vi "Read Pixels and Copy to Display Image New.vi"(0 "fpga interface in":refnum<k20>, 5 "display channel number":i32, 7 "serial channel display parameters":T6[](array[typedef]) {"RAW parameters"."bayer parameters"."blue gain" format="%_4g"; "RAW parameters"."bayer parameters"."green gain" format="%_4g"; "RAW parameters"."bayer parameters"."red gain" format="%_4g"; "RAW parameters"."bayer parameters"."algorithm" items=["Bilinear", "VNG"]; "RAW parameters"."bayer parameters"."pattern" items=["GB", "GR", "BG", "RG"]}, 9 "image metadata":T4, 11 "error in (no error)":errorcluster) -> (4 "fpga interface out":refnum<k20>, 6 "display image":T3, 8 "output cluster":T2, 15 "error out":errorcluster)   [LabVIEW 2026]
uses:
  Types/Serial Channel Display Parameters.ctl
  <vilib>/vision/Image Controls.llb/IMAQ Image.ctl
  Types/RAW Interpretation for Display.ctl
  FPGA/Common/Types/Image Metadata.ctl
  <instrlib>/FlexRIO/CSI-2/v2/Common/Types/LLP Data Type.ctl
  GettingStarted_Common_148X_Host.lvlib
  <instrlib>/FlexRIO/CSI-2/v2/Common/NI CSI-2 API Common v2.lvlib
  FPGA/Common/GettingStarted_Common_148X_FPGA.lvlib
panel:
  in  "Image Metadata and Data":T2 {"RAW parameters"."bayer parameters"."blue gain" format="%_4g"; "RAW parameters"."bayer parameters"."green gain" format="%_4g"; "RAW parameters"."bayer parameters"."red gain" format="%_4g"; "RAW parameters"."bayer parameters"."algorithm" items=["Bilinear", "VNG"]; "RAW parameters"."bayer parameters"."pattern" items=["GB", "GR", "BG", "RG"]}
  out "Array":u8[](array[numeric])
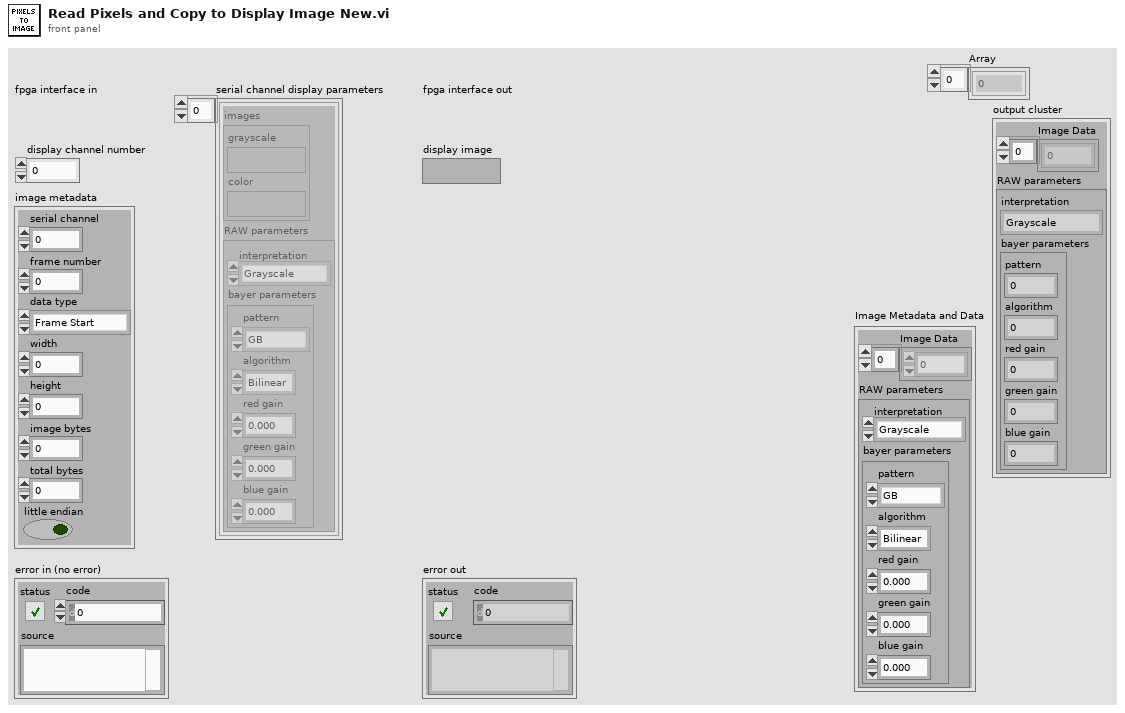
[diagram p1: front panel]
types:
  T1 = typedef "GettingStarted_Common_148X_Host.lvlib/RAW Interpretation for Display.ctl" = enum16{"Grayscale", "Bayer", "RGB", "YUV422", "YUV420", "Legacy YUV420"}
  T2 = cluster{"Image Data":u8[], "RAW parameters":cluster{"interpretation":T1, "bayer parameters":cluster{"pattern":i32, "algorithm":i32, "red gain":dbl, "green gain":dbl, "blue gain":dbl}}}
  T3 = typedef "IMAQ Image.ctl" = refnum<image>
  T4 = typedef "GettingStarted_Common_148X_FPGA.lvlib/Image Metadata.ctl" = cluster{"serial channel":fxp<+,3,3>, "frame number":u16, "data type":T5, "width":u16, "height":u16, "image bytes":u32, "total bytes":u32, "little endian":bool}
  T5 = typedef "NI CSI-2 API Common v2.lvlib/LLP Data Type.ctl" = enum8{"Frame Start", "Frame End", "Line Start", "Line End", "End of Transmission", "Reserved 0", "Reserved 1", "Reserved 2", "Generic Short Packet 1", "Generic Short Packet 2", "Generic Short Packet 3", "Generic Short Packet 4", "Generic Short Packet 5", "Generic Short Packet 6", "Generic Short Packet 7", "Generic Short Packet 8", "Null", "Blanking Data", "Embedded 8-bit non Image Data", "Generic Long Packet 1", "Generic Long Packet 2", "Generic Long Packet 3", "Generic Long Packet 4", "Reserved 3", "YUV420 8-bit", "YUV420 10-bit", "Legacy YUV420 8-bit", "Reserved 4", "YUV420 8-bit Chroma Shifted", "YUV420 10-bit Chroma Shifted", "YUV422 8-bit", "YUV422 10-bit", "RGB444", "RGB555", "RGB565", "RGB666", "RGB888", "Reserved 5", "Reserved 6", "RAW 24", "RAW 6", "RAW 7", "RAW 8", "RAW 10", "RAW 12", "RAW 14", "RAW 16", "RAW 20", "User Defined 8-bit Data 1", "User Defined 8-bit Data 2", "User Defined 8-bit Data 3", "User Defined 8-bit Data 4", "User Defined 8-bit Data 5", "User Defined 8-bit Data 6", "User Defined 8-bit Data 7", "User Defined 8-bit Data 8", "USL Command", "Reserved 7", "Reserved 8", "Reserved 9", "Reserved 10", "Reserved 11", "Reserved 12", "LRTE EPD Spacer"}
  T6 = typedef "GettingStarted_Common_148X_Host.lvlib/Serial Channel Display Parameters.ctl" = cluster{"images":cluster{"grayscale":T3, "color":T3}, "RAW parameters":cluster{"interpretation":T1, "bayer parameters":cluster{"pattern":i32, "algorithm":i32, "red gain":dbl, "green gain":dbl, "blue gain":dbl}}}
  T7 = cluster{"interpretation":T1, "bayer parameters":cluster{"pattern":i32, "algorithm":i32, "red gain":dbl, "green gain":dbl, "blue gain":dbl}}
  T8 = cluster{"pattern":i32, "algorithm":i32, "red gain":dbl, "green gain":dbl, "blue gain":dbl}
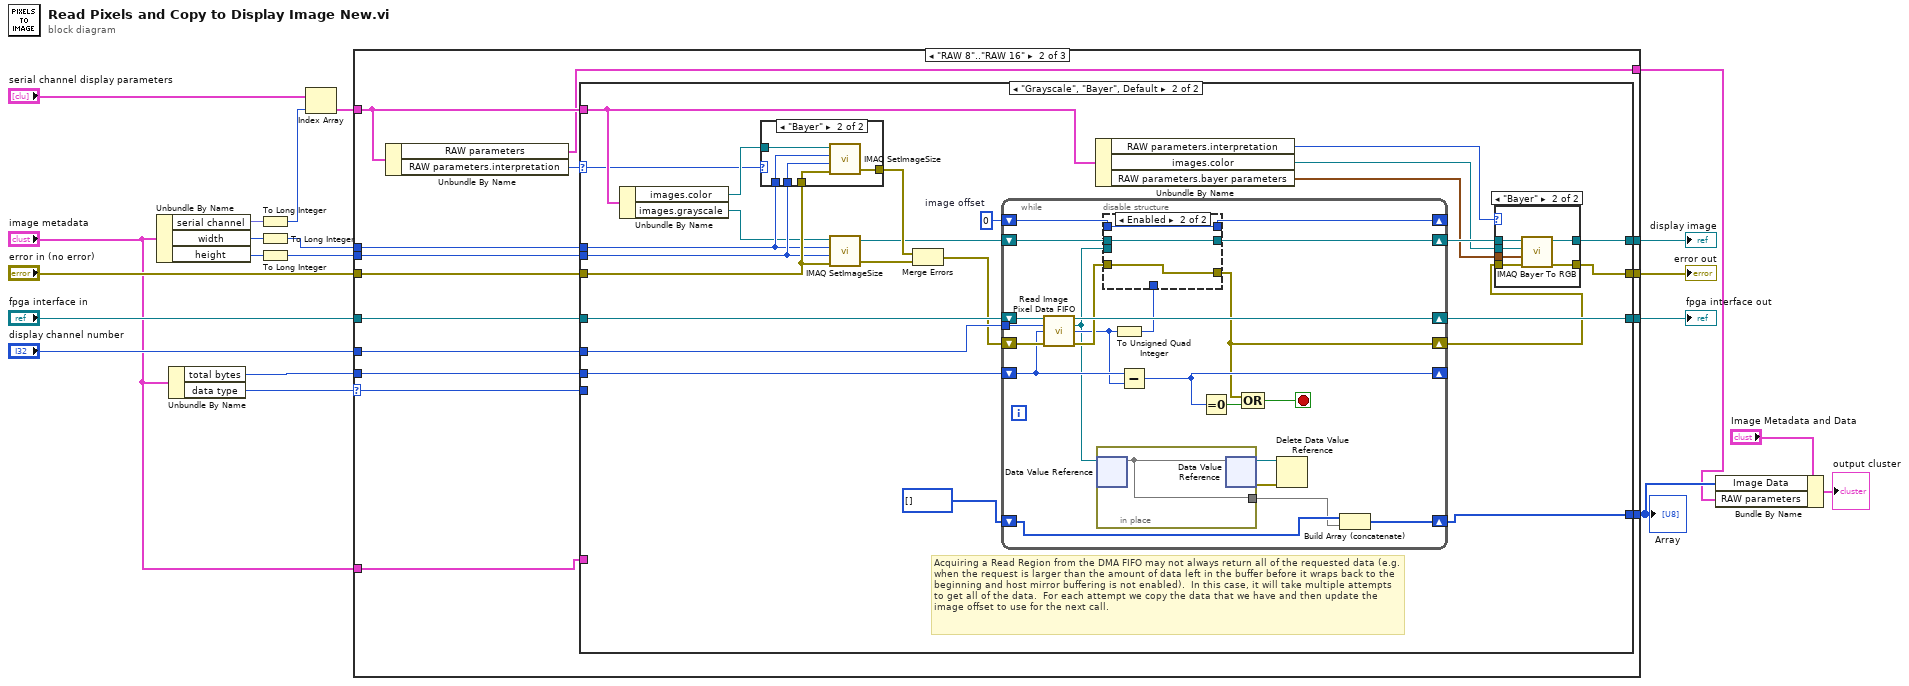
[diagram p0: block diagram]
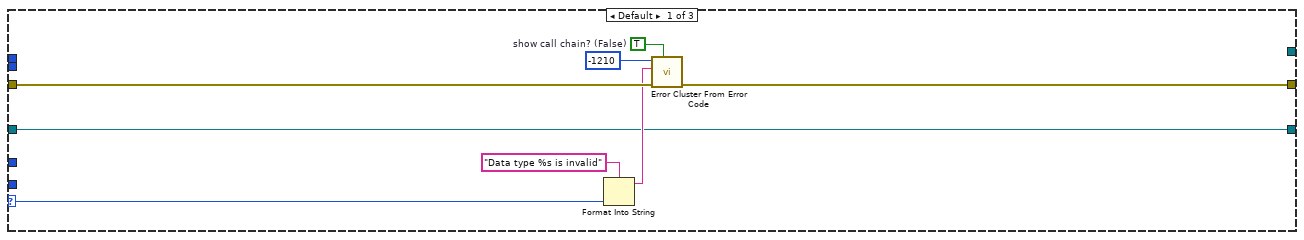
[diagram p2: hidden frame]
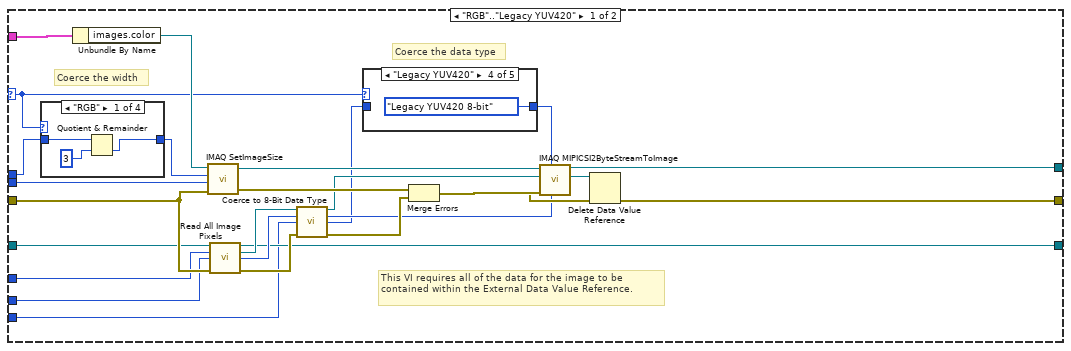
[diagram p3: hidden frame]
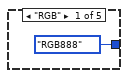
[diagram p4: hidden frame]
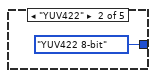
[diagram p5: hidden frame]
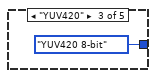
[diagram p6: hidden frame]
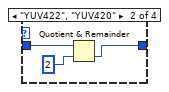
[diagram p8: hidden frame]
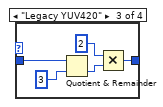
[diagram p9: hidden frame]
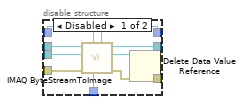
[diagram p12: hidden frame]
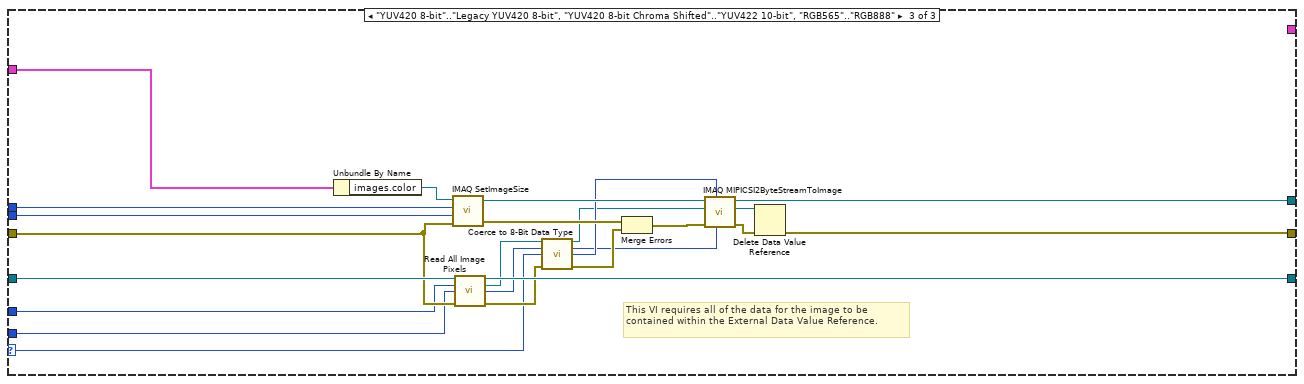
[diagram p14: hidden frame]
diagram:
  n1 = Unbundle By Name("image metadata") -> ("serial channel"=w17:fxp<+,3,3>, "width"=w14:u16, "height"=w15:u16)
  n2 = Unbundle By Name("image metadata") -> ("total bytes"=w20:u32, "data type"=w6:T5)
  n3 = To Long Integer(number=w17) -> (32bit integer=w16:i32)
  n4 = To Long Integer(number=w14) -> (32bit integer=w11:i32)
  n5 = To Long Integer(number=w15) -> (32bit integer=w12:i32)
  n6 = Index Array(array="serial channel display parameters", index=w16) -> (element=w8:T6)
  n7 = case shown="\"RAW 8\"..\"RAW 16\"" w6 {
    selector: w6 -> [w23 w33 w167]
    tunnel: w20 -> [_ w44 w177]
    tunnel: [w22 w43 w179] -> w19
    tunnel: "display channel number" -> [_ w42 w176]
    tunnel: "error in (no error)" -> [w27 w41 w180]
    tunnel: w12 -> [_ w40 w187]
    tunnel: w11 -> [_ w39 w186]
    tunnel: [_ w38 w175] -> w10
    tunnel: [w26 w37 w172] -> w9
    tunnel: w8 -> [_ w35 w184]
    tunnel: "fpga interface in" -> [w22 w36 w183]
    tunnel: [_ w32 _] -> w4
    tunnel: "image metadata" -> [_ w31 _]
    tunnel: [_ w30 _] -> w2
    frame Default {
      w28 = TRUE  # show call chain? (False)
      n8 = Format Into String(format string="Data type %s is invalid" ("error message (\"\")"), w23) -> (resulting string=w24:string)  [unwired: 2 in, 1 out]
      n9 = call <vilib>:"Error Cluster From Error Code.vi"("show call chain? (False)"=w28, "error in (no error)"=w27, "error message (\"\")"=w24, "error code (0)"=-1210) -> ("error out"=w26:errorcluster)  [unwired: 5 in]
    }
    frame "RAW 8".."RAW 16" {
      n10 = Unbundle By Name(w35) -> ("RAW parameters"=w30:T7, "RAW parameters.interpretation"=w34:T1)
      n11 = case shown="\"Grayscale\", \"Bayer\", Default" w34 {
        selector: w34 -> [w47 w91]
        tunnel: w44 -> [w54 w113]
        tunnel: [w58 w111] -> w43
        tunnel: w42 -> [w53 w110]
        tunnel: w41 -> [w59 w109]
        tunnel: w40 -> [w50 w107]
        tunnel: w39 -> [w49 w106]
        tunnel: [w56 w103] -> w38
        tunnel: [w57 w101] -> w37
        tunnel: w35 -> [w52 w96]
        tunnel: w36 -> [w55 w95]
        tunnel: w33 -> [w51 _]
        tunnel: [_ w89] -> w32
        tunnel: w31 -> [_ _]
        frame "RGB".."Legacy YUV420" {
          # "Coerce the data type"
          # "Coerce the width"
          # "This VI requires all of the data for the image to be contained within the External Data Value Reference."
          n12 = case shown="\"RGB\"" w47 {
            tunnel: w49 -> [w78 w81 w87 w88]
            tunnel: [w77 w80 w84 w88] -> w48
            frame "RGB" {
              n13 = Quotient & Remainder(x=w78, y=3) -> (floor(x/y)=w77:i32)  [unwired: 1 out]
            }
            frame "YUV422", "YUV420" {
              n14 = Quotient & Remainder(x=w81, y=2) -> (floor(x/y)=w80:i32)  [unwired: 1 out]
            }
            frame "Legacy YUV420" {
              n15 = Quotient & Remainder(x=w87, y=3) -> (floor(x/y)=w85:i32)  [unwired: 1 out]
              n16 = Multiply(x=2, y=w85) -> (x*y=w84:i32)
            }
            frame Default {
            }
          }
          n17 = Unbundle By Name(w52) -> ("images.color"=w71:T3)
          n18 = call "IMAQ SetImageSize"("error in (no error)"=w59, "Y Resolution"=w50, "X Resolution"=w48, "Image"=w71) -> ("error out"=w69:errorcluster, "Image Out"=w70:T3)  [unwired: 1 in]
          n19 = call "Read All Image Pixels.vi"("fpga inteface in"=w55, "display channel number"=w53, "image bytes"=w54, "error in (no error)"=w59) -> ("fpga interface out"=w58:refnum<k20>, "image pixel data region"=w64:refnum<data-value>, "elements in region"=w63:u32, "error out"=w65:errorcluster)  [unwired: 8 in]
          n20 = call "Coerce to 8-Bit Data Type.vi"("image pixel data region in"=w64, "image bytes in"=w63, "data type in"=w51, "error in (no error)"=w65) -> ("image pixel data region out"=w60:refnum<data-value>, "image bytes out"=w61:u32, "data type out"=w45:T5, "error out"=w62:errorcluster)  [unwired: 8 in]
          n21 = case shown="\"Legacy YUV420\"" w47 {
            tunnel: w45 -> [_ _ _ _ w76]
            tunnel: [LLP_Data_Type."RGB888" ("data type") LLP_Data_Type."YUV422 8-bit" ("data type") LLP_Data_Type."YUV420 8-bit" ("data type") LLP_Data_Type."Legacy YUV420 8-bit" ("data type") w76] -> w46
            frame "RGB" {
            }
            frame "YUV422" {
            }
            frame "YUV420" {
            }
            frame "Legacy YUV420" {
            }
            frame Default {
            }
          }
          n22 = Merge Errors(w69, w62) -> (w68:errorcluster)
          n23 = call "IMAQ MIPICSI2ByteStreamToImage"("Bytes to Copy"=w61, "Format"=w46, "error in (no error)"=w68, "Byte Stream In"=w60, "Image In"=w70) -> ("error out"=w67:errorcluster, "Byte Stream Out"=w66:refnum<data-value>, "Image Out"=w56:T3)  [unwired: 3 in, 1 out]
          n24 = Delete Data Value Reference(data value reference=w66, error in=w67) -> (error out=w57:errorcluster)  [unwired: 1 out]
        }
        frame "Grayscale", "Bayer", Default {
          w92 = u32 0  # image offset
          # "Acquiring a Read Region from the DMA FIFO may not always return all of the requested data (e.g. when the request is larger than the amount of data left in the buffer before it wraps back to the beginning and host mirror buffering is not enabled).  In this case, it will take multiple attempts to get all of the data.  For each attempt we copy the data that we have and then update the image offset to use for the next call."
          n25 = Unbundle By Name(w96) -> ("images.color"=w105:T3, "images.grayscale"=w100:T3)
          n26 = case shown="\"Bayer\"" w91 {
            tunnel: w109 -> [w114 w119]
            tunnel: [w114 w118] -> w108
            tunnel: w105 -> [_ w117]
            tunnel: w107 -> [_ w116]
            tunnel: w106 -> [_ w115]
            frame "Grayscale", Default {
            }
            frame "Bayer" {
              n27 = call "IMAQ SetImageSize"("error in (no error)"=w119, "Y Resolution"=w116, "X Resolution"=w115, "Image"=w117) -> ("error out"=w118:errorcluster)  [unwired: 1 in, 1 out]
            }
          }
          n28 = call "IMAQ SetImageSize"("error in (no error)"=w109, "Y Resolution"=w107, "X Resolution"=w106, "Image"=w100) -> ("error out"=w112:errorcluster, "Image Out"=w94:T3)  [unwired: 1 in]
          n29 = Merge Errors(w108, w112) -> (w93:errorcluster)
          n30 = while {
            tunnel: w110 -> [w139]
            shift-right: [w140] -> w111
            shift-left: w95 -> [w141]
            shift-right: [w128] -> w102
            shift-left: w93 -> [w138]
            shift-right: [w136] -> w104
            shift-left: w94 -> [w137]
            shift-right: [w131] -> _
            shift-left: w113 -> [w133]
            shift-right: [w127] -> _
            shift-left: w92 -> [w126]
            shift-right: [w120] -> w89
            shift-left: u8[] [] -> [w122]
            stop <- w129 stop-if-true
            n31 = call "Read Image Pixel Data FIFO.vi"("fpga inteface in"=w141, "display channel number"=w139, "number of elements"=w133, "error in (no error)"=w138) -> ("fpga interface out"=w140:refnum<k20>, "image pixel data region"=w125:refnum<data-value>, "elements in region"=w132:u32, "error out"=w135:errorcluster)  [unwired: 7 in, 1 out]
            n32 = in-place {
              in-place-border: [w155] -> w121
              n33 = in-place-dvr #1(w125) -> (w155:u8[])  [unwired: 1 out]
              n34 = in-place-dvr #1(w155) -> (w123:refnum<data-value>, w124:errorcluster)
            }
            n35 = To Unsigned Quad Integer(1:w132) -> (0:w134:u64)
            n36 = disable-structure shown="Enabled" {
              disable-tunnel: w137 -> [w151 w154]
              disable-tunnel: [w150 w154] -> w136
              disable-tunnel: w135 -> [w149 w153]
              disable-tunnel: w134 -> [w148 _]
              disable-tunnel: [w145 w153] -> w128
              disable-tunnel: [w144 w152] -> w127
              disable-tunnel: w126 -> [w143 w152]
              disable-tunnel: w125 -> [w142 _]
              frame Disabled {
                n37 = call "IMAQ ByteStreamToImage"("Bytes to Copy"=w148, "Image Byte Offset In"=w143, "error in (no error)"=w149, "Byte Stream In"=w142, "Image In"=w151) -> ("error out"=w146:errorcluster, "Byte Stream Out"=w147:refnum<data-value>, "Image Out"=w150:T3, "Image Byte Offset Out"=w144:u32)  [unwired: 2 in, 1 out]
                n38 = Delete Data Value Reference(data value reference=w147, error in=w146) -> (error out=w145:errorcluster)  [unwired: 1 out]
              }
              frame Enabled {
              }
            }
            n39 = Subtract(x=w133, y=w132) -> (x-y=w131:u32)
            n40 = Equal To 0?(x=w131) -> (x = 0?=w130:bool)
            n41 = Compound Arithmetic op=OR(w128, w130) -> (w129:bool)
            n42 = Delete Data Value Reference(data value reference=w123, error in=w124) -> ()  [unwired: 2 out]
            n43 = Build Array (concatenate)(w122, w121) -> (w120:u8[])
          }
          n44 = Unbundle By Name(w96) -> ("RAW parameters.interpretation"=w97:T1, "images.color"=w98:T3, "RAW parameters.bayer parameters"=w99:T8)
          n45 = case shown="\"Bayer\"" w97 {
            tunnel: w104 -> [w156 w163]
            tunnel: [w156 w162] -> w103
            tunnel: w102 -> [w157 w161]
            tunnel: [w157 w160] -> w101
            tunnel: w98 -> [_ w159]
            tunnel: w99 -> [_ w158]
            frame "Grayscale", Default {
            }
            frame "Bayer" {
              n46 = call "IMAQ Bayer To RGB"("error in (no error)"=w161, "Bayer Parameters"=w158, "Image Dst"=w159, "Image Src"=w163) -> ("error out"=w160:errorcluster, "Image Dst Out"=w162:T3)  [unwired: 6 in]
            }
          }
        }
      }
    }
    frame "YUV420 8-bit".."Legacy YUV420 8-bit", "YUV420 8-bit Chroma Shifted".."YUV422 10-bit", "RGB565".."RGB888" {
      # "This VI requires all of the data for the image to be contained within the External Data Value Reference."
      n47 = Unbundle By Name(w184) -> ("images.color"=w185:T3)
      n48 = call "IMAQ SetImageSize"("error in (no error)"=w180, "Y Resolution"=w187, "X Resolution"=w186, "Image"=w185) -> ("error out"=w181:errorcluster, "Image Out"=w182:T3)  [unwired: 1 in]
      n49 = call "Read All Image Pixels.vi"("fpga inteface in"=w183, "display channel number"=w176, "image bytes"=w177, "error in (no error)"=w180) -> ("fpga interface out"=w179:refnum<k20>, "image pixel data region"=w170:refnum<data-value>, "elements in region"=w169:u32, "error out"=w171:errorcluster)  [unwired: 8 in]
      n50 = call "Coerce to 8-Bit Data Type.vi"("image pixel data region in"=w170, "image bytes in"=w169, "data type in"=w167, "error in (no error)"=w171) -> ("image pixel data region out"=w164:refnum<data-value>, "image bytes out"=w165:u32, "data type out"=w166:T5, "error out"=w168:errorcluster)  [unwired: 8 in]
      n51 = Merge Errors(w181, w168) -> (w178:errorcluster)
      n52 = call "IMAQ MIPICSI2ByteStreamToImage"("Bytes to Copy"=w165, "Format"=w166, "error in (no error)"=w178, "Byte Stream In"=w164, "Image In"=w182) -> ("error out"=w174:errorcluster, "Byte Stream Out"=w173:refnum<data-value>, "Image Out"=w175:T3)  [unwired: 3 in, 1 out]
      n53 = Delete Data Value Reference(data value reference=w173, error in=w174) -> (error out=w172:errorcluster)  [unwired: 1 out]
    }
  }
  "display image" <- w10
  "fpga interface out" <- w19
  "error out" <- w9
  "Array" <- w4
  n54 = Bundle By Name(cluster="Image Metadata and Data", "Image Data"=w4, "RAW parameters"=w2) -> (→"output cluster":T2)
